vi "Autotest.vi"(8 "error in (no error)":errorcluster caption="entrée d'erreur (pas d'erreur)", 11 "Class DIO (Default) en entrée":refnum<class "Class Ana NI.lvclass">) -> (0 "error out":errorcluster caption="sortie d'erreur", 2 "Autotest Ok":bool, 3 "Class DIO (Default) en sortie":refnum<class "Class Ana NI.lvclass">)   [LabVIEW 2020, in "Library Instrument & Equipement.lvlib" / "Library Ana.lvlib" / "Class Ana NI.lvclass"]
uses:
  Class Ana NI.lvclass
  C:/Program Files (x86)/National Instruments/LabVIEW 2020/resource/objmgr/daqmx.rc
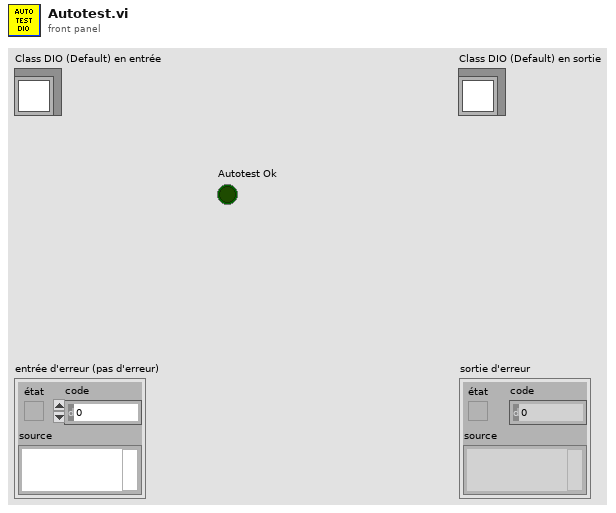
[diagram p1: front panel]
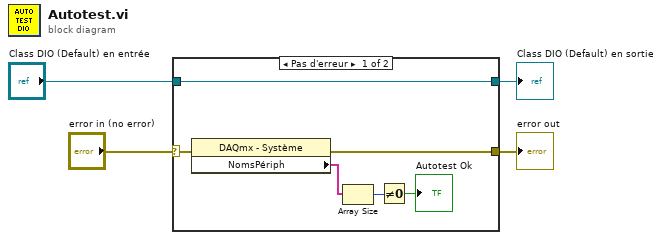
[diagram p0: block diagram]
diagram:
  n1 = case shown="Pas d'erreur" "error in (no error)" {
    selector: "error in (no error)" -> [w9 w12]
    tunnel: [w8 w12] -> w3
    tunnel: [w10 w11] -> w1
    tunnel: "Class DIO (Default) en entrée" -> [w10 w11]
    frame No Error {
      n2 = property class="DAQmx - Système"(error in=w9) -> (error out=w8:errorcluster, "NomsPériph"=w7:tag[])  [unwired: 1 in, 1 out]
      n3 = Array Size(array=w7) -> (size(s)=w5:i32)
      n4 = Not Equal To 0?(x=w5) -> (x != 0?=→"Autotest Ok":bool)
    }
    frame Error {
    }
  }
  "error out" <- w3
  "Class DIO (Default) en sortie" <- w1
